vi "19.1-MovingAverage- Sum.vi"() -> ()   [LabVIEW 2020]
doc: "Uses the Median Filter VI to analyze pulses in the presence of noise. The example generates a pulse contaminated with Gaussian noise and applies a median filter. For comparison purposes, the VI computes the pulse parameters of the filtered pulse."
uses:
  <vilib>/Analysis/2dsp.llb/Real FFT.vi
  <vilib>/Analysis/NI_AALBase.lvlib
  <vilib>/Analysis/NI_AALPro.lvlib
panel:
  out "X[k]H[k]":dbl[](graph)
  out "X[k]":dbl[](graph)
  out "x[n]*h[n]":dbl[](graph)
  out "x[n]":dbl[][](graph)
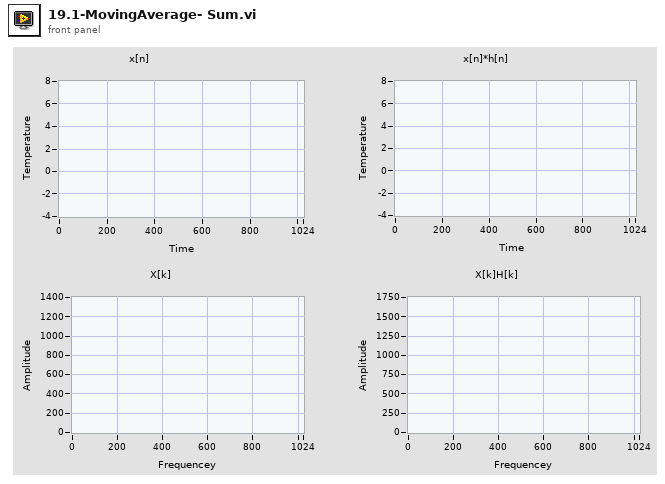
[diagram p1: front panel]
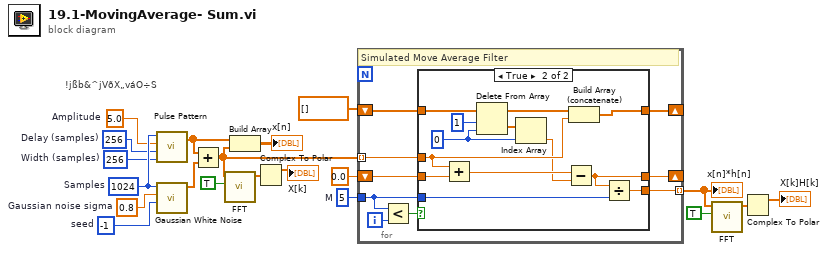
[diagram p0: block diagram]
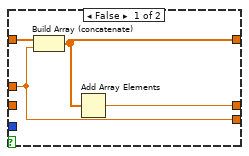
[diagram p2: hidden frame]
diagram:
  w20 = -1  # seed
  w19 = 0.8  # Gaussian noise sigma
  w15 = 256  # Width (samples)
  w16 = 256  # Delay (samples)
  w17 = 5.0  # Amplitude
  w18 = 1024  # Samples
  w14 = 5  # M
  # "!jßb&^jVðX„váO÷S"
  n1 = call <vilib>:"Pulse Pattern.vi"("width"=w15, "delay"=w16, "amplitude"=w17, "samples"=w18) -> ("Pulse Pattern"=w12:dbl[])  [unwired: 1 out]
  n2 = call <vilib>:"Gaussian White Noise.vi"("seed"=w20, "standard deviation"=w19, "samples"=w18) -> ("Gaussian noise pattern"=w13:dbl[])  [unwired: 7 in, 1 out]
  n3 = Add(x=w12, y=w13) -> (x+y=w8:dbl[])
  n4 = call-poly <vilib>:"FFT.vi"("shift?"=TRUE, "X"=w8) -> ("FFT {X}"=w7:cdb[])  [unwired: 8 in, 1 out]
  n5 = Build Array(w12, w8) -> (→"x[n]":dbl[][])
  n6 = Complex To Polar(r * e^(i*theta)=w7) -> (r=→"X[k]":dbl[])  [unwired: 1 out]
  n7 = for {
    tunnel: w14 -> [w21]
    tunnel: w8 -> [w28] mode=indexing
    shift-right: [w27] -> _
    shift-left: dbl[] [] -> [w26]
    shift-right: [w25] -> _
    shift-left: 0.0 -> [w24]
    tunnel: [w23] -> w5 mode=indexing
    i -> [w22]
    # "Simulated Move Average Filter"
    n8 = Less?(x=w21, y=w22) -> (x < y?=w29:bool)
    n9 = case shown="True" w29 {
      tunnel: w28 -> [w30 w42]
      tunnel: [w32 w43] -> w27
      tunnel: w26 -> [w33 w46]
      tunnel: [w31 w36] -> w25
      tunnel: w24 -> [_ w41]
      tunnel: [w30 w34] -> w23
      tunnel: w21 -> [_ w35]
      frame False {
        n10 = Build Array (concatenate)(w33, w30) -> (w32:dbl[])
        n11 = Add Array Elements(numeric array=w32) -> (sum=w31:dbl)
      }
      frame True {
        w38 = 0 ("index")
        n12 = Add(x=w42, y=w41) -> (x+y=w40:dbl)
        n13 = Delete From Array "Delete From Array"(array=w46, length=1, index=w38) -> (deleted portion=w39:dbl[], array with subset deleted=w44:dbl[])
        n14 = Index Array(array=w39, index=w38) -> (element=w37:dbl)
        n15 = Subtract(x=w40, y=w37) -> (x-y=w36:dbl)
        n16 = Build Array (concatenate) "Build Array"(w44, w42) -> (w43:dbl[])
        n17 = Divide(x=w36, y=w35) -> (x/y=w34:dbl)
      }
    }
  }
  "x[n]*h[n]" <- w5
  n18 = call-poly <vilib>:"FFT.vi"("shift?"=TRUE, "X"=w5) -> ("FFT {X}"=w4:cdb[])  [unwired: 8 in, 1 out]
  n19 = Complex To Polar(r * e^(i*theta)=w4) -> (r=→"X[k]H[k]":dbl[])  [unwired: 1 out]
